vi "Доп Код.vi"(1 "C":bool, 2 "B":T2) -> (0 "Result":T1)   [LabVIEW 2017]
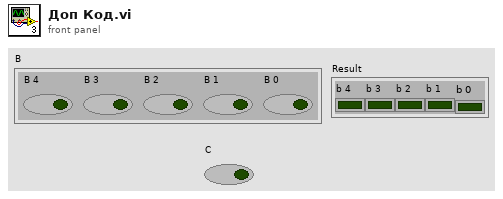
[diagram p1: front panel]
types:
  T1 = cluster{"b 4":bool, "b 3":bool, "b 2":bool, "b 1":bool, "b 0":bool}
  T2 = cluster{"B 4":bool, "B 3":bool, "B 2":bool, "B 1":bool, "B 0":bool}
  T3 = cluster{"SUM":bool, "SUM":bool, "SUM":bool, "SUM":bool, "SUM":bool}
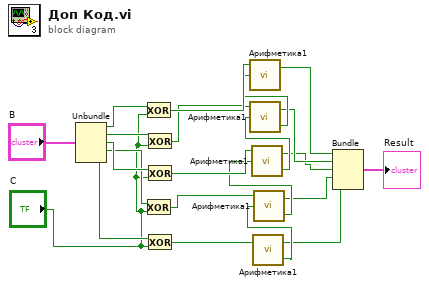
[diagram p0: block diagram]
diagram:
  n1 = Unbundle("B") -> ("B 4"=w21:bool, "B 3"=w20:bool, "B 2"=w19:bool, "B 1"=w18:bool, "B 0"=w17:bool)
  n2 = Exclusive Or(1:"C", 2:w21) -> (0:w15:bool)
  n3 = Exclusive Or(1:"C", 2:w18) -> (0:w11:bool)
  n4 = Exclusive Or(1:"C", 2:w20) -> (0:w13:bool)
  n5 = Exclusive Or(1:"C", 2:w19) -> (0:w12:bool)
  n6 = Exclusive Or(1:"C", 2:w17) -> (0:w10:bool)
  n7 = call "Арифметика1.vi"("A"=w10) -> ("C"=w7:bool, "SUM"=w1:bool)  [unwired: 2 in]
  n8 = call "Арифметика1.vi"("B"=w7, "A"=w11) -> ("C"=w8:bool, "SUM"=w2:bool)  [unwired: 1 in]
  n9 = call "Арифметика1.vi"("B"=w8, "A"=w12) -> ("C"=w9:bool, "SUM"=w3:bool)  [unwired: 1 in]
  n10 = call "Арифметика1.vi"("B"=w9, "A"=w13) -> ("C"=w14:bool, "SUM"=w4:bool)  [unwired: 1 in]
  n11 = call "Арифметика1.vi"("B"=w14, "A"=w15) -> ("SUM"=w5:bool)  [unwired: 1 in, 1 out]
  n12 = Bundle("SUM"=w5, "SUM"=w4, "SUM"=w3, "SUM"=w2, "SUM"=w1) -> (→"Result":T3)  [unwired: 1 in]
